vi "Host.vi"() -> ()   [LabVIEW 2019]
uses:
  TypeDef/TCPMessage.ctl
  <vilib>/Bytelabs/ByteChannelsSetting/ChannelSettingsLib/ChannelsRepos/ChannelsRepoXML/ChannelsRepoXML.lvclass
  bytetcp/TCPLib/TCP_Class/TCP.lvclass
  TypeDef/listChannel.ctl
  TypeDef/ChannelInfo.ctl
  <vilib>/Bytelabs/ByteChannelsSetting/ChannelSettingsLib/ChannelsClasses/ChannelAnalog/AnalogIn/AnalogIn.lvclass
  ByteGSAPIBase/LimsTestStep/acquisitions.ctl
  ByteGSAPIBase/ByteGSAPIBase.lvclass
  <vilib>/Bytelabs/ByteChannelsSetting/ChannelSettingsLib/ChannelsClasses/ChannelBase/ChannelBase.lvclass
  ByteGSAPIBase/TypeDef/Asset.ctl
  ByteGSAPIBase/TypeDef/Step.ctl
  ByteGSAPIBase/UpdateChannelsList/fields.ctl
panel:
  in  "Test":T1={"Step Id"=43, "Test Slug"="T0023", "Duration Seconds"=0.0, "Continous?"=FALSE}
  out "error out":errorcluster
  in  "Stop":bool
  out "Results":T2
  in  "Stop Sequence":bool
  out "Status":string
  out "Raws Readings":cluster{"tag":string, "Value":dbl}[](array[cluster])
  in  "Step  Request":bool
  in  "Channel List":T3[](array[typedef])
  in  "Load":bool
  in  "Configuration":bool
  out "Connected?":bool
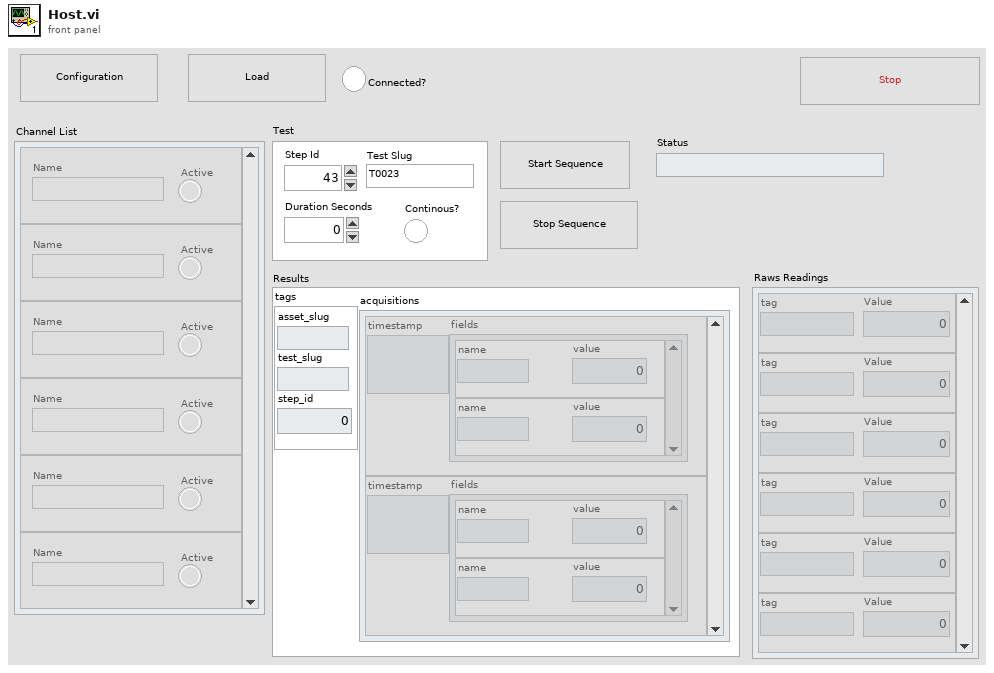
[diagram p1: front panel]
types:
  T1 = cluster{"Step Id":u32, "Test Slug":string, "Duration Seconds":dbl, "Continous?":bool}
  T2 = typedef "ByteQXWebAPI.lvlib/ByteGSAPIBase.lvclass/acquisitions.ctl" = cluster{"tags":cluster{"step_id":i32, "test_slug":string, "asset_slug":string}, "acquisitions":cluster{"timestamp":string, "fields":cluster{"name":string, "value":dbl}[]}[]}
  T3 = typedef "listChannel.ctl" = cluster{"Name":string, "Active":bool}
  T4 = typedef "TCPMessage.ctl" = cluster{"Message":string, "Data":variant}
  T5 = cluster{"Event Registration Refnum":refnum<event-registration>, "ChannelsRepoBase out":refnum<class "ChannelsRepoXML.lvclass">, "TCP_Class":refnum<class "TCP.lvclass">, "Data":variant, "Stauts":string, "notifier out":refnum<notifier>}
  T6 = typedef "ChannelInfo.ctl" = cluster{"Tag":string, "HW Resource":string, "Raw":dbl}
  T7 = typedef "ByteQXWebAPI.lvlib/ByteGSAPIBase.lvclass/fields.ctl" = cluster{"asset_slug":string, "fields":string[]}
  T8 = cluster{"Channel List":T3[], "Test":cluster{"Step Id":u32, "Test Slug":string, "Duration Seconds":dbl, "Continous?":bool}}
  T9 = map{i32, map{string, refnum<class "ChannelBase.lvclass">}}
  T10 = typedef "ByteQXWebAPI.lvlib/ByteGSAPIBase.lvclass/Step.ctl" = cluster{"id":i32, "descrizione":string, "prova":cluster{"slug":string}, "assets":T11[], "criterio_accettazione":string, "valore_criterio_accettazione_max":dbl, "valore_criterio_accettazione_min":dbl, "udm_criterio_accettazione":string, "duration_prova":string, "udm_duration_prova":string, "valore_prova":dbl, "ordine":i32, "user":i32, "link_automation":string, "instruction_automation":string, "data_completamento_checklist":timestamp, "outcome":bool, "step_type":string, "channels":string[]}
  T11 = typedef "ByteQXWebAPI.lvlib/ByteGSAPIBase.lvclass/Asset.ctl" = cluster{"descrizione":string, "slug":string, "id":i32}
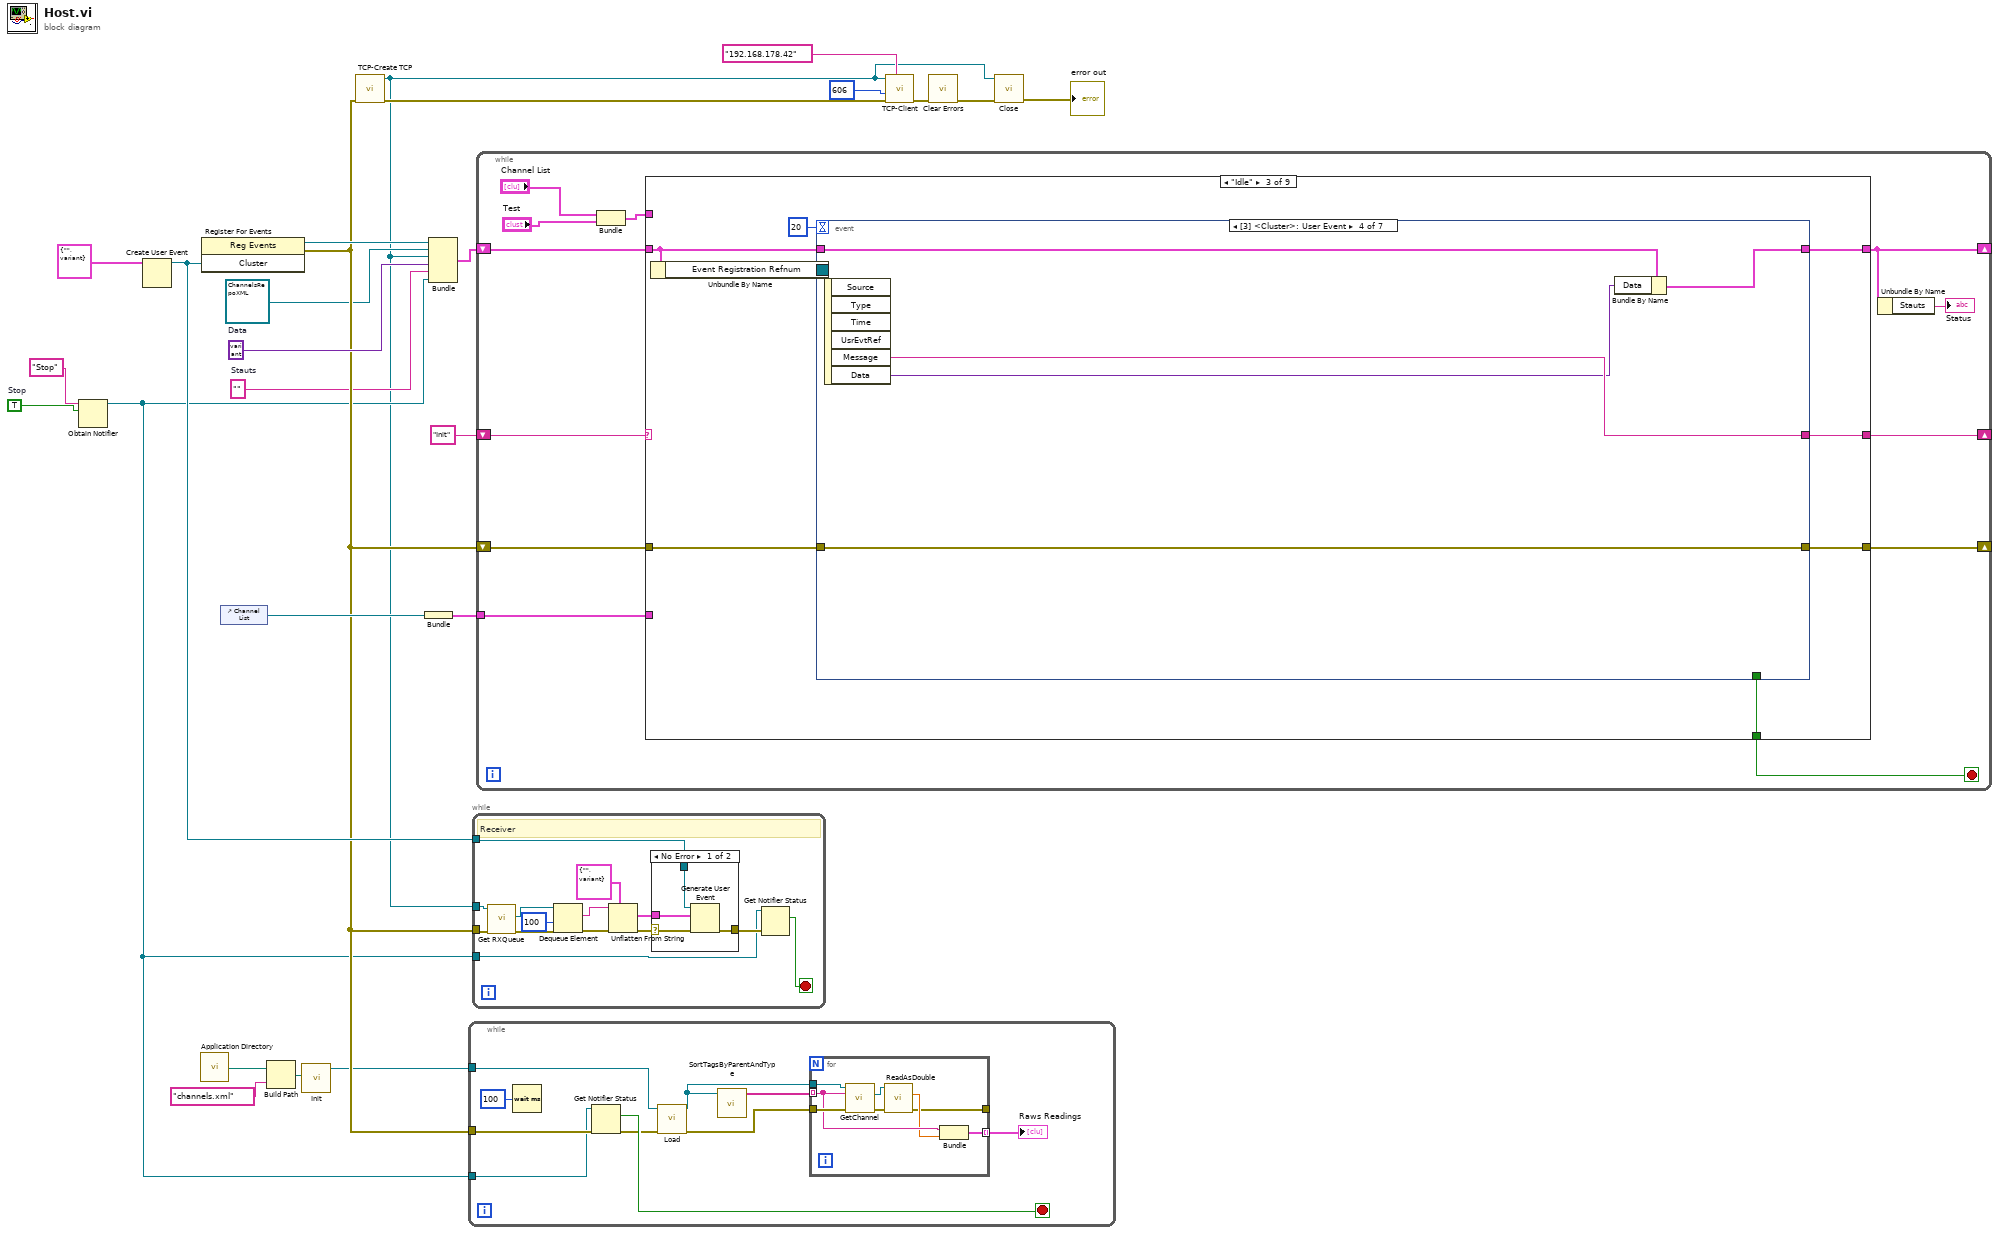
[diagram p0: block diagram]
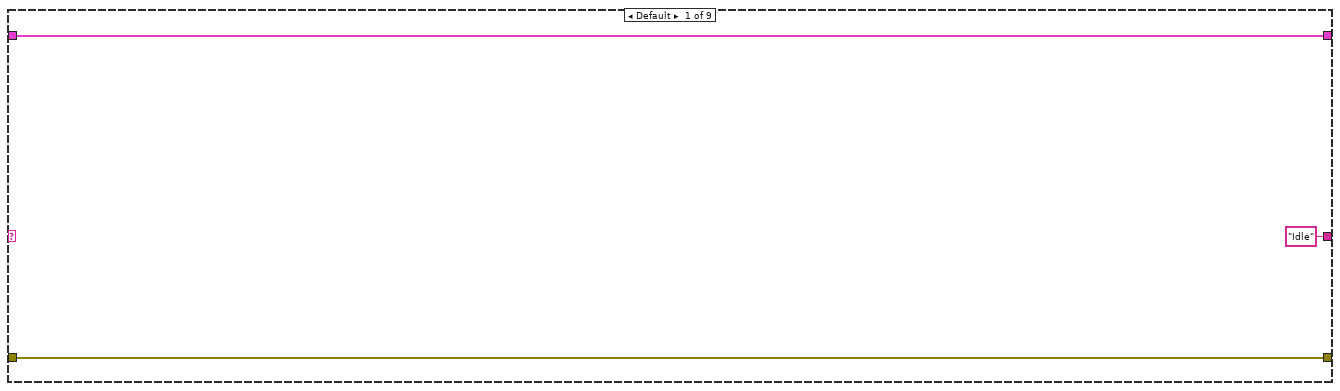
[diagram p2: hidden frame]
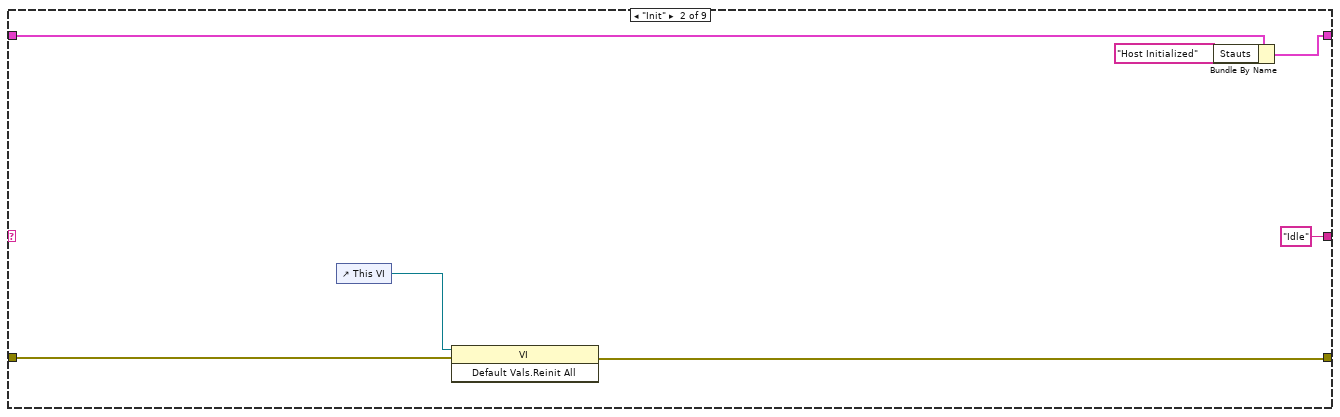
[diagram p3: hidden frame]
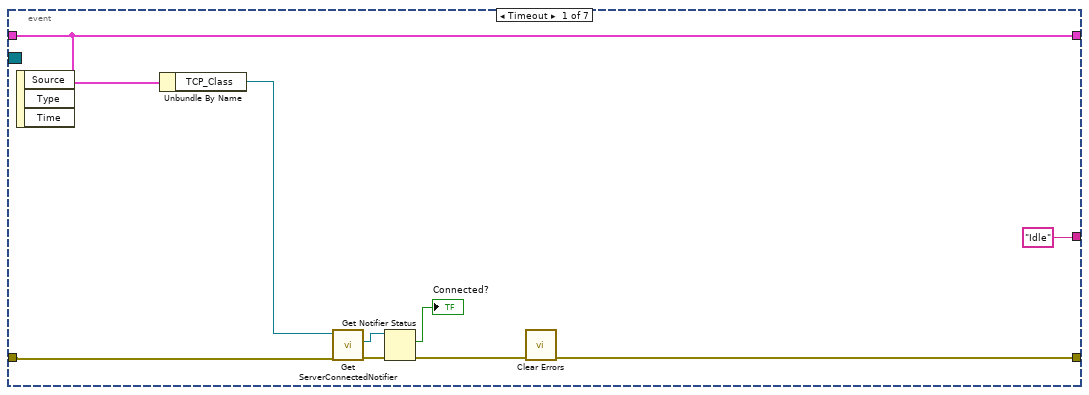
[diagram p4: hidden frame]
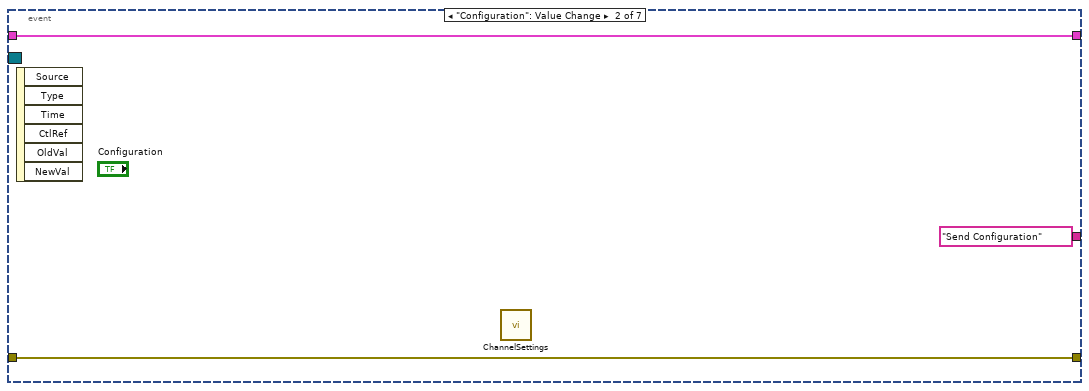
[diagram p5: hidden frame]
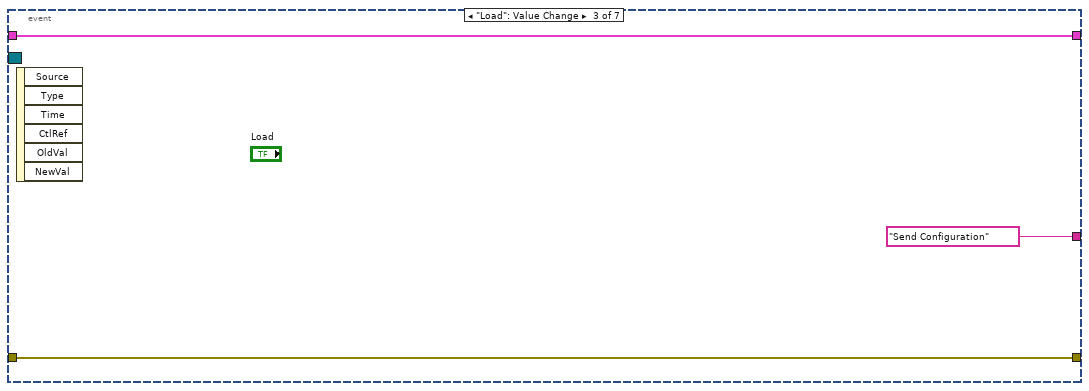
[diagram p6: hidden frame]
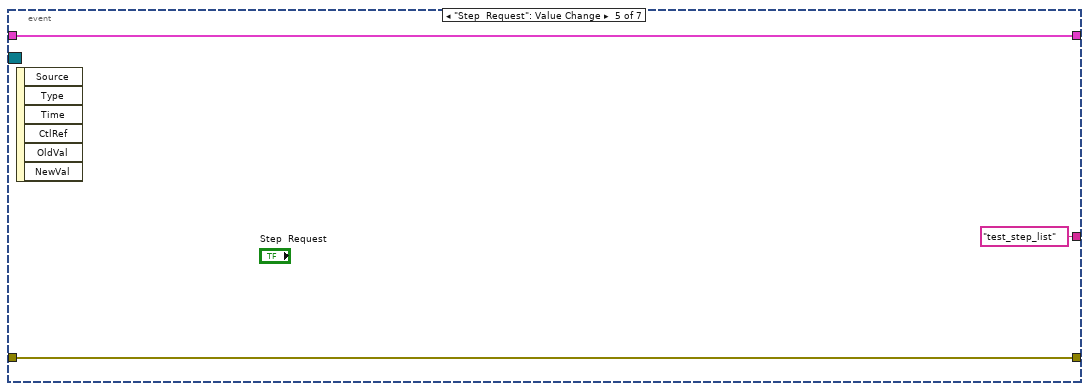
[diagram p7: hidden frame]
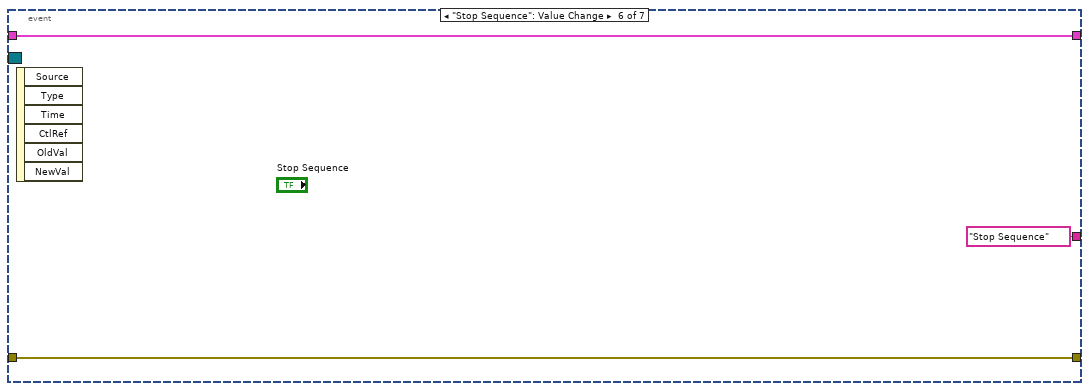
[diagram p8: hidden frame]
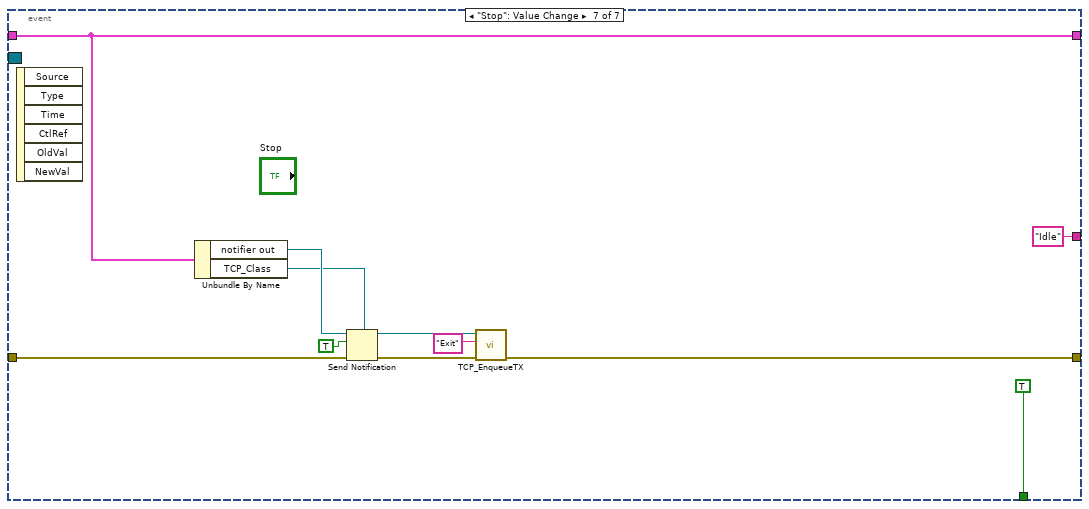
[diagram p9: hidden frame]
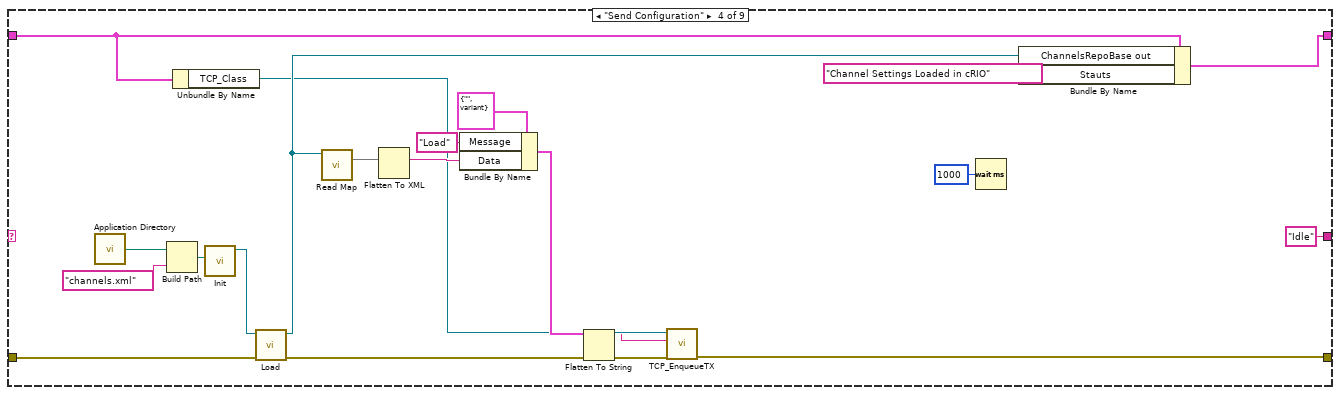
[diagram p10: hidden frame]
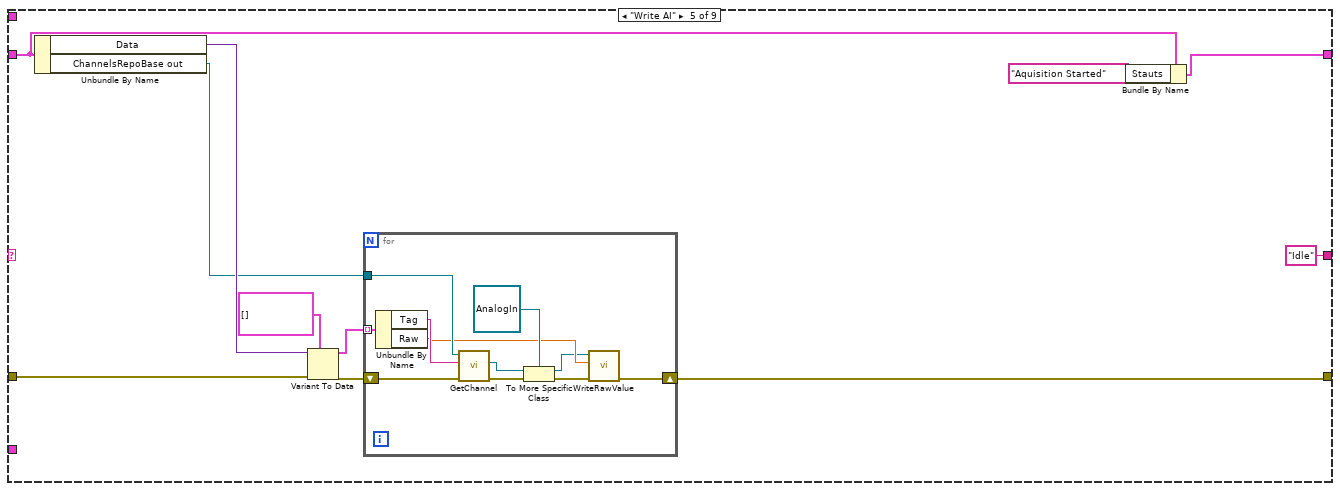
[diagram p11: hidden frame]
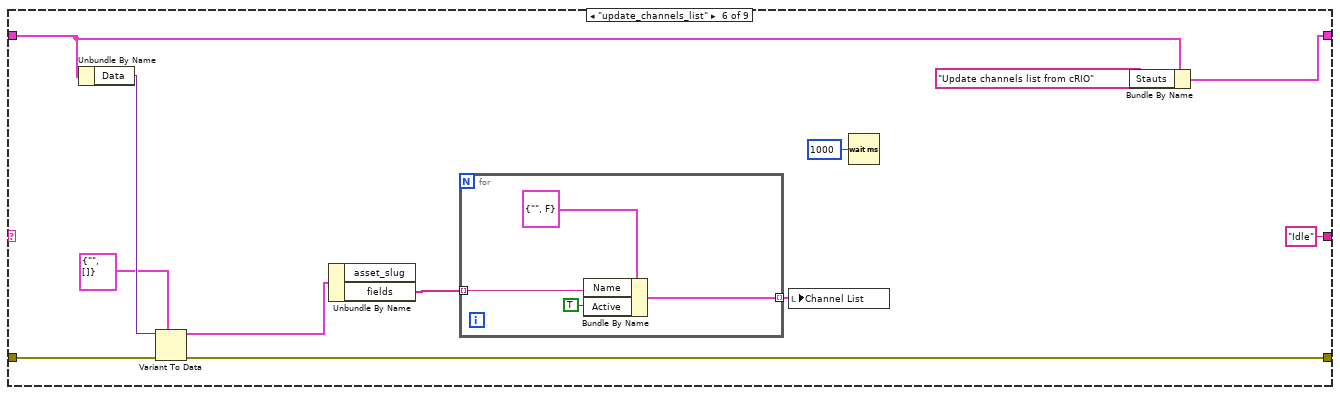
[diagram p12: hidden frame]
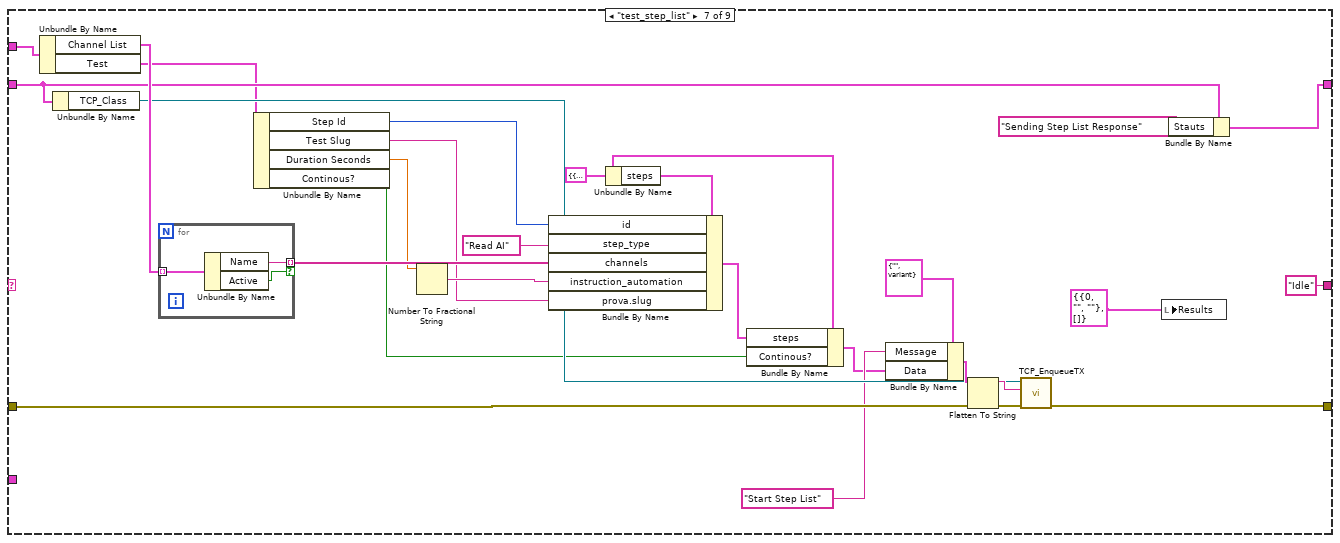
[diagram p13: hidden frame]
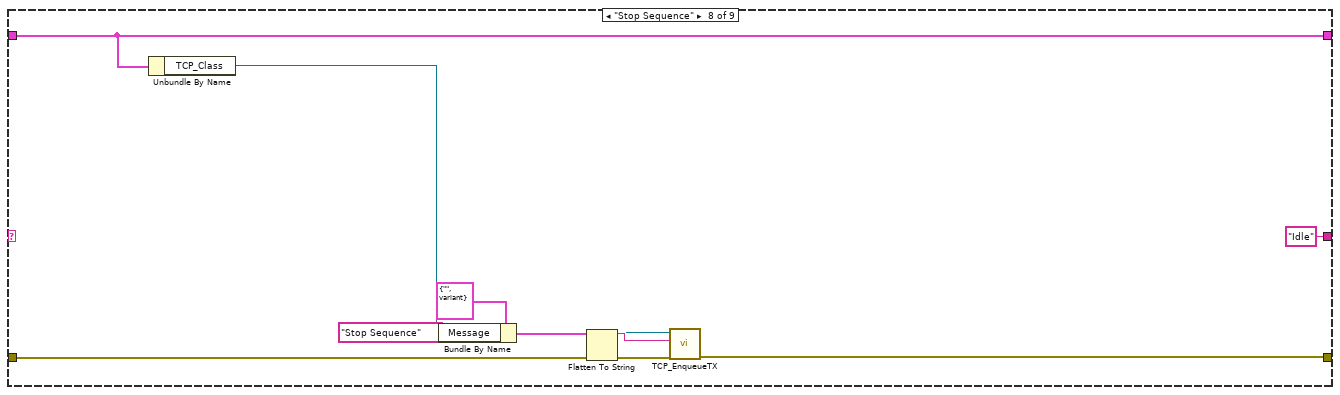
[diagram p14: hidden frame]
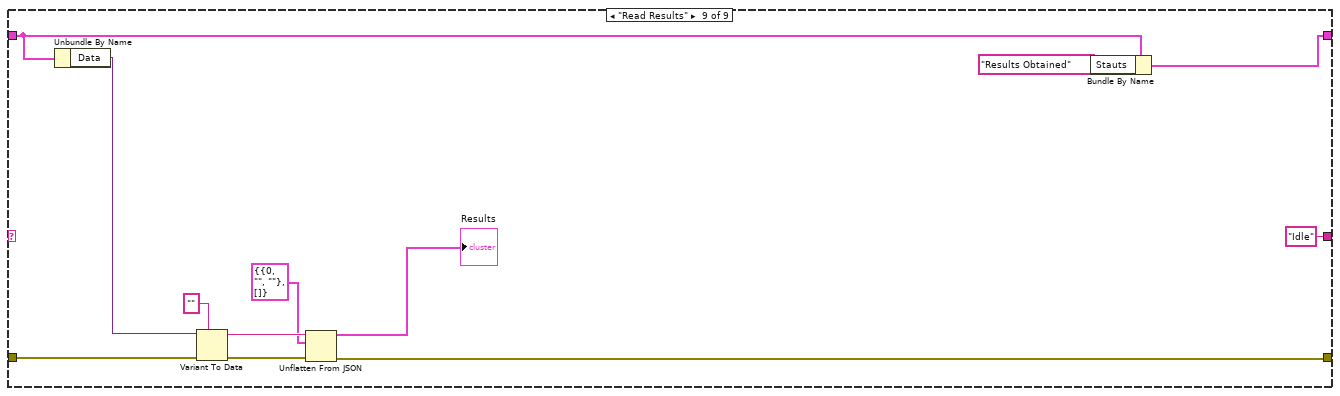
[diagram p15: hidden frame]
diagram:
  w11 = TRUE  # Stop
  w12 = ""  # Stauts
  w17 = variant  # Data
  n1 = Obtain Notifier(name (unnamed)="Stop", notification data type=w11) -> (notifier out=w9:refnum<notifier>)  [unwired: 2 in, 2 out]
  n2 = Create User Event(user event datatype=T4 {"Message"="", "Data"=variant} ("Cluster")) -> (user event=w22:refnum<user-event>)  [unwired: 1 in, 1 out]
  n3 = call <vilib>:"Application Directory.vi"() -> ("Application Directory"=w3:path)
  n4 = register-events(w22) -> (reference out=w21:refnum<event-registration>, error out=w14:errorcluster)  [unwired: 2 in]
  n5 = control-ref of="Channel List"() -> (w16:refnum<vi>)
  n6 = Build Path(base path=w3, name or relative path="channels.xml") -> (appended path=w4:path)
  n7 = call <vilib>:"Init.vi"("XML file path"=w4) -> ("ChannelsRepoXML out"=w1:refnum<class "ChannelsRepoXML.lvclass">)  [unwired: 10 in]
  n8 = call "TCP-Create TCP.vi"("error in (no error)"=w14) -> ("error out"=w23:errorcluster, "TCP_Class"=w8:refnum<class "TCP.lvclass">)  [unwired: 8 in, 1 out]
  n9 = Bundle("Channel List"=w16) -> (w15:cluster{"Channel List":refnum<vi>})  [unwired: 1 in]
  n10 = Bundle("Event Registration Refnum"=w21, "ChannelsRepoBase out"=refnum<class "ChannelsRepoXML.lvclass"> refnum, "TCP_Class"=w8, "Data"=w17, "Stauts"=w12, "notifier out"=w9) -> (w20:T5)  [unwired: 1 in]
  n11 = while {
    tunnel: w14 -> [w31]
    tunnel: w9 -> [w30]
    tunnel: w1 -> [w27]
    stop <- w29 stop-if-true
    n12 = Wait (ms)(milliseconds to wait=u32 100) -> ()  [unwired: 1 out]
    n13 = Get Notifier Status(notifier=w30, error in (no error)=w31) -> (current notification=w29:bool, error out=w28:errorcluster)  [unwired: 3 out]
    n14 = call <vilib>:"Load.vi"("error in (no error)"=w28, "ChannelsRepoBase in"=w27) -> ("error out"=w33:errorcluster, "ChannelsRepoBase out"=w32:refnum<class "ChannelsRepoXML.lvclass">)  [unwired: 7 in, 1 out]
    n15 = call <vilib>:"SortTagsByParentAndType.vi"("ChannelsRepoBase in"=w32) -> ("sorted tags"=w35:string[])  [unwired: 8 in, 2 out]
    n16 = for {
      tunnel: w33 -> [w43]
      tunnel: w35 -> [w40] mode=indexing
      tunnel: [w38] -> w34 mode=indexing
      tunnel: [w37] -> _
      tunnel: w32 -> [w36]
      n17 = call <vilib>:"GetChannel.vi"("error in (no error)"=w43, "tag"=w40, "ChannelsRepoBase in"=w36) -> ("error out"=w42:errorcluster, "channel"=w41:refnum<class "ChannelBase.lvclass">)  [unwired: 5 in, 2 out]
      n18 = call-dynamic "ReadAsDouble.vi"("error in (no error)"=w42, "ChannelBase in"=w41) -> ("error out"=w37:errorcluster, "Value"=w39:dbl)  [unwired: 7 in, 1 out]
      n19 = Bundle("tag"=w40, "Value"=w39) -> (w38:cluster{"tag":string, "Value":dbl})  [unwired: 1 in]
    }
    "Raws Readings" <- w34
  }
  n20 = while {
    tunnel: w8 -> [w52]
    tunnel: w14 -> [w53]
    tunnel: w22 -> [w56]
    tunnel: w9 -> [w46]
    stop <- w45 stop-if-true
    # "Receiver"
    n21 = call-dynamic "Get RXQueue.vi"("error in (no error)"=w53, "TCP in"=w52) -> ("error out"=w51:errorcluster, "RX"=w48:refnum<queue>)  [unwired: 7 in, 1 out]
    n22 = Dequeue Element(queue=w48, timeout in ms (-1)=100, error in (no error)=w51) -> (element=w49:string, error out=w50:errorcluster)  [unwired: 2 out]
    n23 = Unflatten From String(type=T4 {"Message"="", "Data"=variant} ("Cluster"), binary string=w49, error in (no error)=w50) -> (value=w55:T4, error out=w57:errorcluster)  [unwired: 2 in, 1 out]
    n24 = case shown="No Error" w57 {
      selector: w57 -> [w61 _]
      tunnel: w56 -> [w60 _]
      tunnel: w55 -> [w59 _]
      tunnel: [w58 _] -> w47
      frame No Error {
        n25 = Generate User Event(user event=w60, event data cluster=w59, error in=w61) -> (error out=w58:errorcluster)  [unwired: 1 in, 1 out]
      }
      frame Error {
      }
    }
    n26 = Get Notifier Status(notifier=w46, error in (no error)=w47) -> (current notification=w45:bool)  [unwired: 4 out]
  }
  n27 = while {
    shift-right: [w65] -> _
    shift-left: w20 -> [w71]
    shift-right: [w72] -> _
    shift-left: "Init" -> [w73]
    shift-right: [w69] -> _
    shift-left: w14 -> [w70]
    tunnel: w15 -> [w66]
    stop <- w63 stop-if-true
    n28 = Bundle("Channel List"="Channel List", "Test"="Test") -> (w67:T8)  [unwired: 1 in]
    n29 = case shown="\"Idle\"" w73 {
      tunnel: ["Idle" "Idle" w88 "Idle" "Idle" ("Message") "Idle" ("Message") "Idle" ("Message") "Idle" ("Message") "Idle" ("Message")] -> w72
      tunnel: w71 -> [w76 w79 w86 w136 w151 w175 w200 w218 w231]
      tunnel: [w76 w77 w87 w135 w150 w173 w199 w218 w229] -> w65
      tunnel: w70 -> [w74 w82 w90 w138 w154 w182 w213 w221 w235]
      tunnel: [w74 w80 w89 w132 w153 w177 w203 w220 w234] -> w69
      tunnel: w67 -> [_ _ _ _ _ _ w211 _ _]
      tunnel: w66 -> [_ _ _ _ _ _ _ _ _]
      tunnel: [_ _ w84 _ _ _ _ _ _] -> w63
      frame Default {
      }
      frame "Init" {
        n30 = control-ref of="This VI"() -> (w81:refnum<vi>)
        n31 = invoke class="VI" method="Default Vals.Reinit All"(reference=w81, error in=w82) -> (error out=w80:errorcluster)  [unwired: 1 in, 2 out]
        n32 = Bundle By Name(cluster=w79, "Stauts"="Host Initialized") -> (w77:T5)
      }
      frame "Idle" {
        n33 = Unbundle By Name(w86) -> ("Event Registration Refnum"=w85:refnum<event-registration>)
        n34 = event shown="[3] <Cluster>: User Event" {
          selector: w85 -> [_ _ _ _ _ _ _]
          dyn-events: _ -> [_ _ _ _ _ _ _]
          timeout: 20 -> [_ _ _ _ _ _ _]
          tunnel: w86 -> [w94 w103 w106 w110 w114 w116 w125]
          tunnel: w90 -> [w96 w102 w104 w107 w113 w117 w123]
          tunnel: [w92 w102 w104 w107 w113 w117 w120] -> w89
          tunnel: ["Idle" "Send Configuration" "Send Configuration" w111 "test_step_list" ("Message") "Stop Sequence" ("Message") "Idle" ("Message")] -> w88
          tunnel: [w94 w103 w106 w109 w114 w116 w125] -> w87
          tunnel: [_ _ _ _ _ _ TRUE] -> w84
          event Timeout {
            n35 = event-data() -> ()  [unwired: 1 in, 3 out]
            n36 = Unbundle By Name(w94) -> ("TCP_Class"=w97:refnum<class "TCP.lvclass">)
            n37 = call-dynamic "Get ServerConnectedNotifier.vi"("error in (no error)"=w96, "TCP in"=w97) -> ("error out"=w98:errorcluster, "IsServerConnected?"=w99:refnum<notifier>)  [unwired: 7 in, 1 out]
            n38 = Get Notifier Status(notifier=w99, error in (no error)=w98) -> (current notification=→"Connected?":bool, error out=w93:errorcluster)  [unwired: 3 out]
            n39 = call <vilib>:"Clear Errors.vi"("error in (no error)"=w93) -> ("error out"=w92:errorcluster)  [unwired: 5 in, 1 out]
          }
          event "Configuration": Value Change {
            n40 = event-data() -> ()  [unwired: 1 in, 6 out]
            n41 = call "ChannelSettings.vi"() -> ()  [unwired: 12 in]
          }
          event "Load": Value Change {
            n42 = event-data() -> ()  [unwired: 1 in, 6 out]
          }
          event User Event {
            n43 = event-data() -> ("Message"=w111:string, "Data"=w108:variant)  [unwired: 1 in, 4 out]
            n44 = Bundle By Name(cluster=w110, "Data"=w108) -> (w109:T5)
          }
          event "Step  Request": Value Change {
            n45 = event-data() -> ()  [unwired: 1 in, 6 out]
          }
          event "Stop Sequence": Value Change {
            n46 = event-data() -> ()  [unwired: 1 in, 6 out]
          }
          event "Stop": Value Change {
            n47 = event-data() -> ()  [unwired: 1 in, 6 out]
            n48 = Unbundle By Name(w125) -> ("notifier out"=w124:refnum<notifier>, "TCP_Class"=w119:refnum<class "TCP.lvclass">)
            n49 = Send Notification(notification=TRUE, notifier=w124, error in (no error)=w123) -> (error out=w121:errorcluster)  [unwired: 1 out]
            n50 = call-dynamic "TCP_EnqueueTX.vi"("error in (no error)"=w121, "Msg to Transmit"="Exit", "TCP in"=w119) -> ("error out"=w120:errorcluster)  [unwired: 7 in, 1 out]
          }
        }
      }
      frame "Send Configuration" {
        n51 = call <vilib>:"Application Directory.vi"() -> ("Application Directory"=w142:path)
        n52 = Build Path(base path=w142, name or relative path="channels.xml") -> (appended path=w141:path)
        n53 = Unbundle By Name(w136) -> ("TCP_Class"=w131:refnum<class "TCP.lvclass">)
        n54 = call <vilib>:"Init.vi"("XML file path"=w141) -> ("ChannelsRepoXML out"=w140:refnum<class "ChannelsRepoXML.lvclass">)  [unwired: 10 in]
        n55 = call <vilib>:"Load.vi"("error in (no error)"=w138, "ChannelsRepoBase in"=w140) -> ("error out"=w137:errorcluster, "ChannelsRepoBase out"=w134:refnum<class "ChannelsRepoXML.lvclass">)  [unwired: 7 in, 1 out]
        n56 = call <vilib>:"Read Map.vi"("ChannelsRepoBase in"=w134) -> ("Map"=w145:T9)  [unwired: 9 in, 1 out]
        n57 = Flatten To XML(anything=w145) -> (xml string=w144:string)
        n58 = Bundle By Name(cluster=T4 {"Message"="", "Data"=variant} ("Cluster"), "Message"="Load", "Data"=w144) -> (w143:T4)
        n59 = Flatten To String(anything=w143, error in (no error)=w137) -> (data string=w130:string, error out=w133:errorcluster)  [unwired: 2 in, 1 out]
        n60 = call-dynamic "TCP_EnqueueTX.vi"("error in (no error)"=w133, "Msg to Transmit"=w130, "TCP in"=w131) -> ("error out"=w132:errorcluster)  [unwired: 7 in, 1 out]
        n61 = Wait (ms)(milliseconds to wait=u32 1000) -> ()  [unwired: 1 out]
        n62 = Bundle By Name(cluster=w136, "ChannelsRepoBase out"=w134, "Stauts"="Channel Settings Loaded in cRIO") -> (w135:T5)
      }
      frame "Write AI" {
        n63 = Unbundle By Name(w151) -> ("Data"=w159:variant, "ChannelsRepoBase out"=w156:refnum<class "ChannelsRepoXML.lvclass">)
        n64 = Variant To Data(error in=w154, type=T6[] [] ("Array"), Variant=w159) -> (data=w155:T6[], error out=w157:errorcluster)
        n65 = for {
          tunnel: w156 -> [w168]
          shift-right: [w162] -> w153
          shift-left: w157 -> [w170]
          tunnel: w155 -> [w160] mode=indexing
          n66 = Unbundle By Name(w160) -> ("Tag"=w169:string, "Raw"=w164:dbl)
          n67 = call <vilib>:"GetChannel.vi"("error in (no error)"=w170, "tag"=w169, "ChannelsRepoBase in"=w168) -> ("error out"=w167:errorcluster, "channel"=w161:refnum<class "ChannelBase.lvclass">)  [unwired: 5 in, 2 out]
          n68 = To More Specific Class(target class=refnum<class "AnalogIn.lvclass"> refnum ("ChannelSettings.lvlib:ChannelsClasses.lvlib:AnalogIn.lvclass"), reference=w161, error in=w167) -> (specific class reference=w163:refnum<class "AnalogIn.lvclass">, error out=w165:errorcluster)
          n69 = call <vilib>:"WriteRawValue.vi"("error in (no error)"=w165, "Raw value"=w164, "AnalogIn in"=w163) -> ("error out"=w162:errorcluster)  [unwired: 7 in, 1 out]
        }
        n70 = Bundle By Name(cluster=w151, "Stauts"="Aquisition Started") -> (w150:T5)
      }
      frame "update_channels_list" {
        n71 = Unbundle By Name(w175) -> ("Data"=w181:variant)
        n72 = Variant To Data(error in=w182, type=T7 {"asset_slug"="", "fields"=[]} ("Channels"), Variant=w181) -> (data=w176:T7, error out=w177:errorcluster)
        n73 = Unbundle By Name(w176) -> ("fields"=w179:string[])  [unwired: 1 out]
        n74 = for {
          tunnel: w179 -> [w185] mode=indexing
          tunnel: [w183] -> w178 mode=indexing
          n75 = Bundle By Name(cluster=T3 {"Name"="", "Active"=FALSE} ("Cluster"), "Name"=w185, "Active"=TRUE) -> (w183:T3)
        }
        n76 = local write "Channel List"(w178) -> ()
        n77 = Wait (ms)(milliseconds to wait=u32 1000) -> ()  [unwired: 1 out]
        n78 = Bundle By Name(cluster=w175, "Stauts"="Update channels list from cRIO") -> (w173:T5)
      }
      frame "test_step_list" {
        w190 = cluster{"steps":T10, "Continous?":bool} {"steps"={"id"=0, "descrizione"="", "prova"={"slug"=""}, "assets"=[], "criterio_accettazione"="", "valore_criterio_accettazione_max"=0.0, "valore_criterio_accettazione_min"=0.0, "udm_criterio_accettazione"="", "duration_prova"="", "udm_duration_prova"="", "valore_prova"=0.0, "ordine"=0, "user"=0, "link_automation"="", "instruction_automation"="", "data_completamento_checklist"=timestamp(0 s since 1904-01-01), "outcome"=FALSE, "step_type"="", "channels"=[]}, "Continous?"=FALSE}
        n79 = Unbundle By Name(w211) -> ("Channel List"=w210:T3[], "Test"=w193:T1)
        n80 = Unbundle By Name(w200) -> ("TCP_Class"=w202:refnum<class "TCP.lvclass">)
        n81 = for {
          tunnel: w210 -> [w216] mode=indexing
          tunnel: [w215] -> w209 mode=indexing if=w214
          n82 = Unbundle By Name(w216) -> ("Name"=w215:string, "Active"=w214:bool)
        }
        n83 = Unbundle By Name(w193) -> ("Step Id"=w195:u32, "Test Slug"=w194:string, "Duration Seconds"=w192:dbl, "Continous?"=w188:bool)
        n84 = Number To Fractional String(number=w192) -> (F-format string=w197:string)  [unwired: 3 in]
        n85 = Unbundle By Name(w190) -> ("steps"=w191:T10)
        n86 = Bundle By Name(cluster=w191, "id"=w195, "step_type"="Read AI", "channels"=w209, "instruction_automation"=w197, "prova.slug"=w194) -> (w189:T10)
        n87 = Bundle By Name(cluster=w190, "steps"=w189, "Continous?"=w188) -> (w187:cluster{"steps":T10, "Continous?":bool})
        n88 = Bundle By Name(cluster=T4 {"Message"="", "Data"=variant} ("Cluster"), "Message"="Start Step List", "Data"=w187) -> (w205:T4)
        n89 = Flatten To String(anything=w205, error in (no error)=w213) -> (data string=w204:string, error out=w206:errorcluster)  [unwired: 2 in, 1 out]
        n90 = call-dynamic "TCP_EnqueueTX.vi"("error in (no error)"=w206, "Msg to Transmit"=w204, "TCP in"=w202) -> ("error out"=w203:errorcluster)  [unwired: 7 in, 1 out]
        n91 = local write "Results"(T2 {"tags"={"step_id"=0, "test_slug"="", "asset_slug"=""}, "acquisitions"=[]}) -> ()
        n92 = Bundle By Name(cluster=w200, "Stauts"="Sending Step List Response") -> (w199:T5)
      }
      frame "Stop Sequence" {
        n93 = Unbundle By Name(w218) -> ("TCP_Class"=w217:refnum<class "TCP.lvclass">)
        n94 = Bundle By Name(cluster=T4 {"Message"="", "Data"=variant} ("Cluster"), "Message"="Stop Sequence") -> (w224:T4)
        n95 = Flatten To String(anything=w224, error in (no error)=w221) -> (data string=w222:string, error out=w223:errorcluster)  [unwired: 2 in, 1 out]
        n96 = call-dynamic "TCP_EnqueueTX.vi"("error in (no error)"=w223, "Msg to Transmit"=w222, "TCP in"=w217) -> ("error out"=w220:errorcluster)  [unwired: 7 in, 1 out]
      }
      frame "Read Results" {
        n97 = Unbundle By Name(w231) -> ("Data"=w233:variant)
        n98 = Variant To Data(error in=w235, type="", Variant=w233) -> (data=w236:string, error out=w238:errorcluster)
        n99 = Unflatten From JSON(JSON string=w236, type and defaults=T2 {"tags"={"step_id"=0, "test_slug"="", "asset_slug"=""}, "acquisitions"=[]}, error in (no error)=w238) -> (value=→"Results":T2, error out=w234:errorcluster)  [unwired: 4 in]
        n100 = Bundle By Name(cluster=w231, "Stauts"="Results Obtained") -> (w229:T5)
      }
    }
    n101 = Unbundle By Name(w65) -> ("Stauts"=→"Status":string)
  }
  n102 = call "TCP-Client.vi"("IP address"="192.168.178.42", "error in (no error)"=w23, "TXport"=u16 606 ("port"), "TCP.lvclass"=w8) -> ("error out"=w6:errorcluster)  [unwired: 7 in]
  n103 = call <vilib>:"Clear Errors.vi"("error in (no error)"=w6) -> ("error out"=w5:errorcluster)  [unwired: 5 in, 1 out]
  n104 = call-dynamic "Close.vi"("error in (no error)"=w5, "TCP in"=w8) -> ("error out"=→"error out":errorcluster)  [unwired: 5 in, 4 out]
